vi "del Create Event.vi"(9 "Event":refnum<class "Event.lvclass">, 10 "Self Event Alias":string, 11 "Base Queue in":refnum<class "Base Queue.lvclass">) -> (3 "Base Queue out":refnum<class "Base Queue.lvclass">)   [LabVIEW 2021, in "jettl.lvlib" / "Base Queue.lvlib" / "Base Queue.lvclass"]
uses:
  Base Queue.lvclass
  Base Queue.lvclass/Base Queue.ctl
  Error/Error.lvlib
  Msg Strategy/Msg Strategy.lvclass
  Event/Event.lvclass
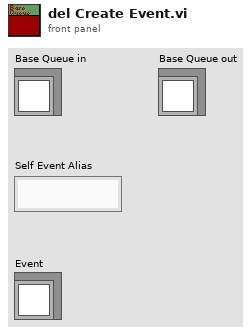
[diagram p1: front panel]
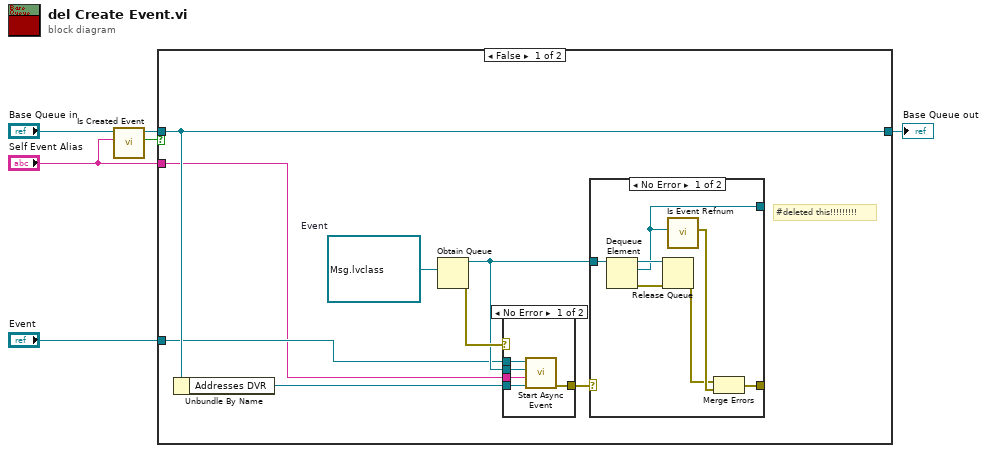
[diagram p0: block diagram]
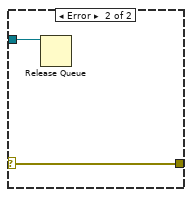
[diagram p2: hidden frame]
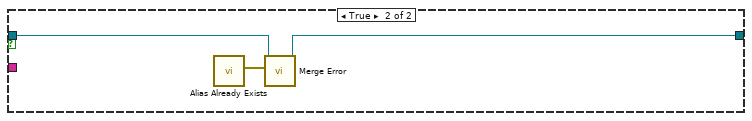
[diagram p4: hidden frame]
diagram:
  n1 = call-dynamic "Is Created Event.vi"("Created Event Alias"="Self Event Alias", "Base Queue in"="Base Queue in") -> ("Is Created Event?"=w2:bool, "Base Queue out"=w1:refnum<class "Base Queue.lvclass">)  [unwired: 8 in]
  n2 = case shown="False" w2 {
    tunnel: "Event" -> [w11 _]
    tunnel: w1 -> [w13 w32]
    tunnel: "Self Event Alias" -> [w7 _]
    tunnel: [w13 w31] -> w5
    frame False {
      w9 = refnum<data-value> refnum  # Event
      # "#deleted this!!!!!!!!!"
      n3 = Unbundle By Name(w13) -> ("Addresses DVR"=w8:refnum<data-value>)
      n4 = Obtain Queue(element data type=w9) -> (queue out=w12:refnum<queue>, error out=w14:errorcluster)  [unwired: 4 in, 1 out]
      n5 = case shown="No Error" w14 {
        selector: w14 -> [_ w29]
        tunnel: [w27 w29] -> w10
        tunnel: w11 -> [w28 _]
        tunnel: w12 -> [w25 _]
        tunnel: w7 -> [w24 _]
        tunnel: w8 -> [w26 _]
        frame No Error {
          n6 = call "Start Async Event.vi"("Queue Mailbox"=w26, "Self Event Alias"=w24, "Queue of Self Event"=w25, "Event"=w28) -> ("error out"=w27:errorcluster)  [unwired: 7 in]
        }
        frame Error {
        }
      }
      n7 = case shown="No Error" w10 {
        selector: w10 -> [_ w23]
        tunnel: [w19 w23] -> _
        tunnel: w12 -> [w18 w22]
        tunnel: [w17 _] -> _
        frame No Error {
          n8 = Dequeue Element(queue=w18) -> (queue out=w20:refnum<queue>, element=w17:refnum<data-value>, error out=w21:errorcluster)  [unwired: 2 in, 1 out]
          n9 = Release Queue(queue=w20, error in (no error)=w21) -> (error out=w15:errorcluster)  [unwired: 1 in, 2 out]
          n10 = call "Is Event Refnum.vi"("Self Event"=w17) -> ("Error"=w16:errorcluster)  [unwired: 10 in]
          n11 = Merge Errors(w15, w16) -> (w19:errorcluster)
        }
        frame Error {
          n12 = Release Queue(queue=w22) -> ()  [unwired: 2 in, 3 out]
        }
      }
    }
    frame True {
      n13 = call "Alias Already Exists.vi"() -> ("Error"=w30:errorcluster)  [unwired: 11 in]
      n14 = call-dynamic "Merge Error.vi"("Error"=w30, "Base Queue in"=w32) -> ("Base Queue out"=w31:refnum<class "Base Queue.lvclass">)  [unwired: 9 in]
    }
  }
  "Base Queue out" <- w5
